vi "Read BoolText.vi"(9 "Boolean in":refnum<class "Boolean.lvclass">) -> (3 "Boolean out":refnum<class "Boolean.lvclass">, 4 "BoolText":refnum<class "Text.lvclass">)   [LabVIEW 2014, in "Boolean.lvclass"]
uses:
  Boolean.lvclass
  Text/Text.lvclass
  Boolean.lvclass/Boolean.ctl
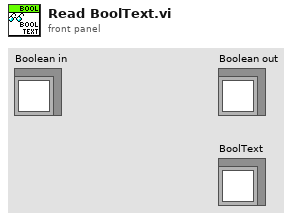
[diagram p1: front panel]
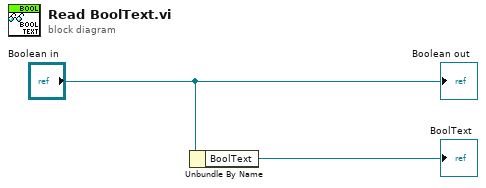
[diagram p0: block diagram]
diagram:
  n1 = Unbundle By Name("Boolean in") -> ("BoolText"=→"BoolText":refnum<class "Text.lvclass">)
  "Boolean out" <- "Boolean in"
